vi "Set Folders.vi"(8 "error in (no error)":errorcluster, 9 "Local folder":path, 10 "Calibration folder":path, 11 "SigMan in":refnum<class "SignalManager.lvclass">) -> (0 "error out":errorcluster, 3 "SigMan out":refnum<class "SignalManager.lvclass">)   [LabVIEW 2015, in "SignalManager.lvclass"]
uses:
  SignalManager.lvclass
  SignalManager.lvclass/SignalManager.ctl
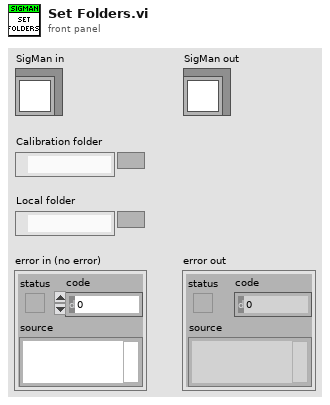
[diagram p1: front panel]
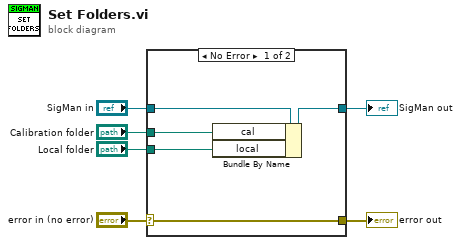
[diagram p0: block diagram]
diagram:
  n1 = case shown="No Error" "error in (no error)" {
    selector: "error in (no error)" -> [w10 w13]
    tunnel: [w10 w13] -> w5
    tunnel: [w9 w12] -> w3
    tunnel: "SigMan in" -> [w11 w12]
    tunnel: "Calibration folder" -> [w8 _]
    tunnel: "Local folder" -> [w7 _]
    frame No Error {
      n2 = Bundle By Name(cluster=w11, "cal"=w8, "local"=w7) -> (w9:refnum<class "SignalManager.lvclass">)
    }
    frame Error {
    }
  }
  "error out" <- w5
  "SigMan out" <- w3
